vi "INI Read write bool.vi"(5 "key":string, 7 "section":string, 8 "error in":errorcluster, 9 "Default":bool, 10 "Boolean in":bool, 11 "Read|Write":T1) -> (0 "error out":errorcluster, 2 "Boolean out":bool)   [LabVIEW 2010]
doc: "This .vi reads/writes a boolean to the config file. During Write, \"bool in\" is passed to \"bool out\""
uses:
  Read write mode.ctl
  <vilib>/Utility/config.llb/Read Key (Boolean).vi
  <vilib>/Utility/config.llb/Write Key (Boolean).vi
  <vilib>/Utility/config.llb/NI_LVConfig.lvlib
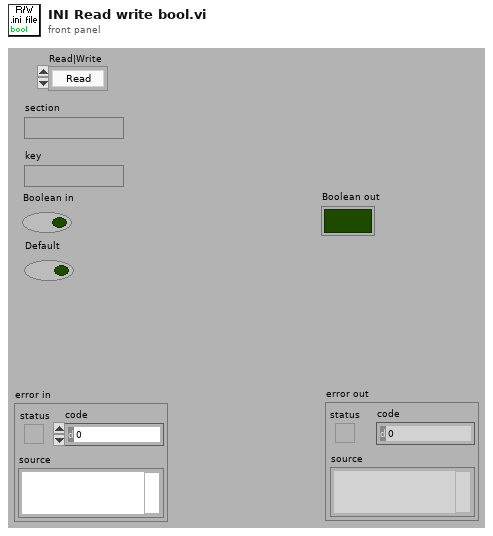
[diagram p1: front panel]
types:
  T1 = typedef "Read write mode.ctl" = enum16{"Read", "Write"}
  T2 = typedef "Semaphore RefNum" = refnum<k1>
  T3 = typedef "NI_LVConfig.lvlib/Config Data RefNum.ctl" = refnum<k1>
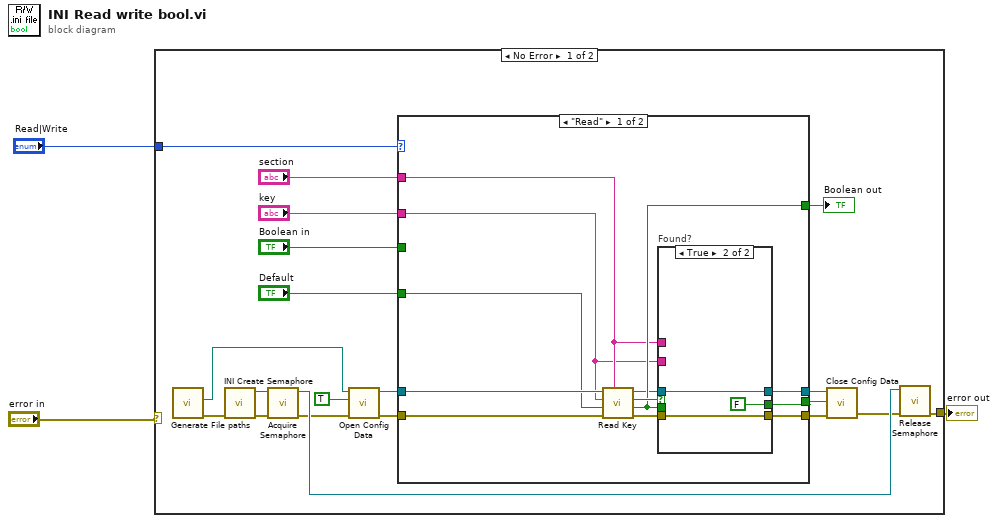
[diagram p0: block diagram]
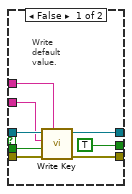
[diagram p2: hidden frame]
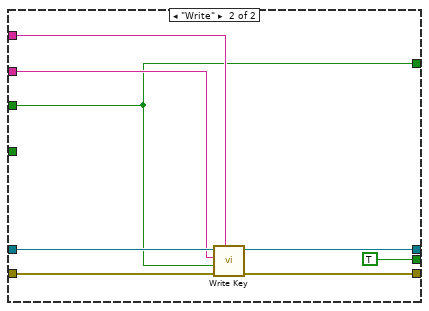
[diagram p3: hidden frame]
diagram:
  n1 = case shown="No Error" "error in" {
    selector: "error in" -> [_ w55]
    tunnel: "Read|Write" -> [w23 _]
    tunnel: [w8 w55] -> w1
    frame No Error {
      n2 = call "Generate File paths.vi"() -> ("error out"=w5:errorcluster, ".ini path"=w4:path)  [unwired: 1 in, 9 out]
      n3 = call "INI Create Semaphore.vi"("error in"=w5) -> ("error out"=w7:errorcluster, "semaphore"=w6:T2)  [unwired: 1 in, 4 out]
      n4 = call <vilib>:"Acquire Semaphore.vi"("error in (no error)"=w7, "semaphore"=w6) -> ("error out"=w10:errorcluster, "semaphore out"=w11:T2)  [unwired: 1 in, 3 out]
      n5 = call <vilib>:"Open Config Data.vi"("error in (no error)"=w10, "create file if necessary (T)"=TRUE ("create file if necessary? (T)"), "configuration file path"=w4) -> ("error out"=w18:errorcluster, "refnum"=w21:T3)  [unwired: 6 in, 1 out]
      n6 = case shown="\"Read\"" w23 {
        tunnel: [w31 w53] -> w20
        tunnel: w21 -> [w35 w54]
        tunnel: [w27 w52] -> w19
        tunnel: w18 -> [w34 w51]
        tunnel: "section" -> [w26 w50]
        tunnel: "key" -> [w25 w49]
        tunnel: [w29 w47] -> w15
        tunnel: "Boolean in" -> [_ w47]
        tunnel: [w24 TRUE ("write configuration file? (T)")] -> w13
        tunnel: "Default" -> [w33 _]
        frame "Read" {
          n7 = call-poly <vilib>:"Read Key.vi"("section"=w26, "error in (no error)"=w34, "default value"=w33, "key"=w25, "refnum"=w35) -> ("error out"=w32:errorcluster, "value"=w29:bool, "found?"=w30:bool, "refnum out"=w28:T3)  [unwired: 3 out]
          n8 = case "Found?" shown="True" w30 {
            tunnel: w32 -> [w43 w46]
            tunnel: [w42 w46] -> w31
            tunnel: w29 -> [w41 _]
            tunnel: w28 -> [w40 w45]
            tunnel: [w39 w45] -> w27
            tunnel: w26 -> [w38 _]
            tunnel: w25 -> [w37 _]
            tunnel: [TRUE ("write configuration file? (T)") FALSE ("write configuration file? (T)")] -> w24
            frame False {
              # "Write\ndefault\nvalue."
              n9 = call-poly <vilib>:"Write Key.vi"("section"=w38, "error in (no error)"=w43, "value"=w41, "key"=w37, "refnum"=w40) -> ("error out"=w42:errorcluster, "refnum out"=w39:T3)  [unwired: 5 out]
            }
            frame True {
            }
          }
        }
        frame "Write" {
          n10 = call-poly <vilib>:"Write Key.vi"("section"=w50, "error in (no error)"=w51, "value"=w47, "key"=w49, "refnum"=w54) -> ("error out"=w53:errorcluster, "refnum out"=w52:T3)  [unwired: 5 out]
        }
      }
      "Boolean out" <- w15
      n11 = call <vilib>:"Close Config Data.vi"("error in (no error)"=w20, "write file if changed (T)"=w13, "refnum"=w19) -> ("error out"=w9:errorcluster)  [unwired: 8 out]
      n12 = call <vilib>:"Release Semaphore.vi"("error in (no error)"=w9, "semaphore"=w11) -> ("error out"=w8:errorcluster)  [unwired: 5 out]
    }
    frame Error {
    }
  }
  "error out" <- w1
